vi "Read CamSession.vi"(8 "error in (no error)":errorcluster, 11 "FakeCamera in":refnum<class "MoveDataFile.lvclass">) -> (0 "error out":errorcluster, 2 "CamSession":string, 3 "FakeCamera out":refnum<class "MoveDataFile.lvclass">)   [LabVIEW 2011, in "MoveDataFile.lvclass"]
uses:
  MoveDataFile.lvclass
  MoveDataFile.lvclass/MoveDataFile.ctl
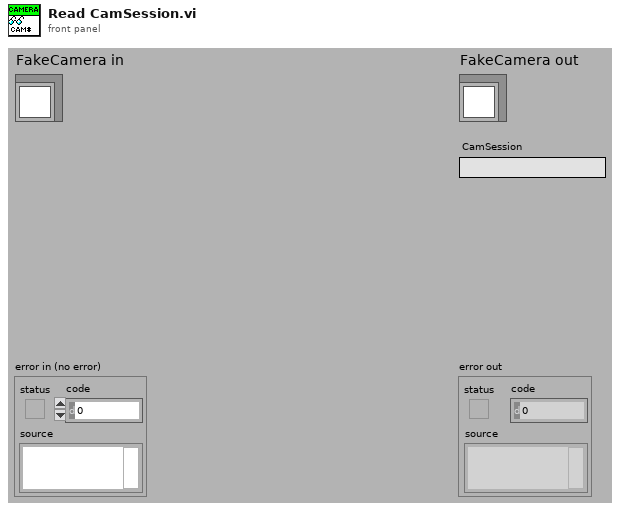
[diagram p1: front panel]
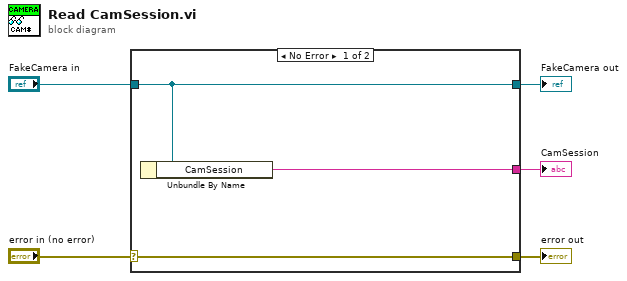
[diagram p0: block diagram]
diagram:
  n1 = case shown="No Error" "error in (no error)" {
    selector: "error in (no error)" -> [w8 w9]
    tunnel: [w8 w9] -> w4
    tunnel: [w7 w10] -> w2
    tunnel: "FakeCamera in" -> [w7 w10]
    tunnel: [w6 _] -> w1
    frame No Error {
      n2 = Unbundle By Name(w7) -> ("CamSession"=w6:string)
    }
    frame Error {
    }
  }
  "error out" <- w4
  "FakeCamera out" <- w2
  "CamSession" <- w1
